vi "GSE 350 Extract Component Data.vi"(6 "Negative Number":bool, 8 "Error In":errorcluster, 10 "Title":string="Tare Weight", 11 "Data Stream":string) -> (0 "Error Out":errorcluster, 2 "Weight":dbl, 3 "Array":string[](array[string]))   [LabVIEW 2019]
uses:
  <vilib>/Utility/error.llb/whitespace.ctl
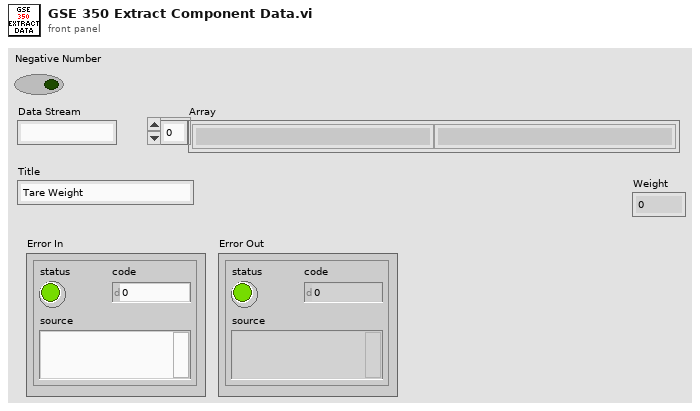
[diagram p1: front panel]
types:
  T1 = typedef "whitespace.ctl" = u16
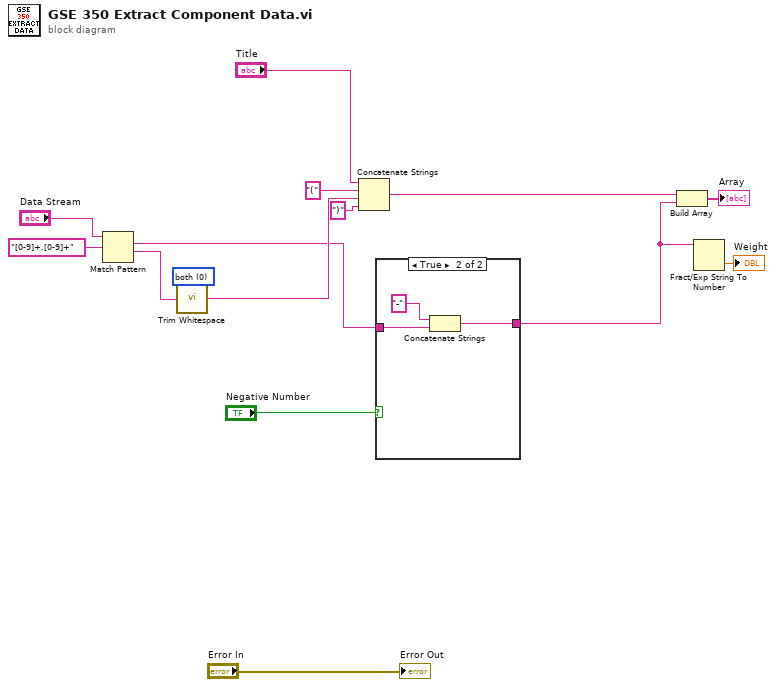
[diagram p0: block diagram]
diagram:
  w14 = T1 0 items=["both", "start of string", "end of string"] ("location (both)")
  n1 = Match Pattern(string="Data Stream", regular expression="[0-9]+.[0-9]+") -> (match substring=w2:string, after substring=w13:string)  [unwired: 1 in, 2 out]
  n2 = call <vilib>:"Trim Whitespace.vi"("string"=w13, "location (both)"=w14) -> ("trimmed string"=w15:string)
  n3 = Concatenate Strings("Title", "(" ("string"), w15, ")" ("string")) -> (w11:string)
  n4 = case shown="True" "Negative Number" {
    tunnel: w2 -> [w16 w19]
    tunnel: [w16 w17] -> w1
    frame False {
    }
    frame True {
      n5 = Concatenate Strings("-" ("string"), w19) -> (w17:string)
    }
  }
  n6 = Build Array(w11, w1) -> (→"Array":string[])
  n7 = Fract/Exp String To Number(string=w1) -> (number=→"Weight":dbl)  [unwired: 3 in, 1 out]
  "Error Out" <- "Error In"
